vi "UsrProfiles-Save new profile.vi"() -> ()   [LabVIEW 2020]
uses:
  Typedefs/Which path.ctl
  Globals/gl_UsrProfiles globals.vi
panel:
  out "error out":errorcluster
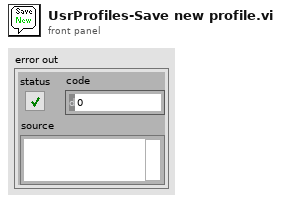
[diagram p1: front panel]
types:
  T1 = typedef "Which path.ctl" = enum16{"Configuration Files", "Calibration Files", "Images", "Setup.ini", "Loaded User profile.ini", "User's-Previous session.ini", "New user profile.ini", "Selected User profile.ini", "User profiles folder", "Power meter scaling.txt", "FOV Cal.ini", "Calibration.ini"}
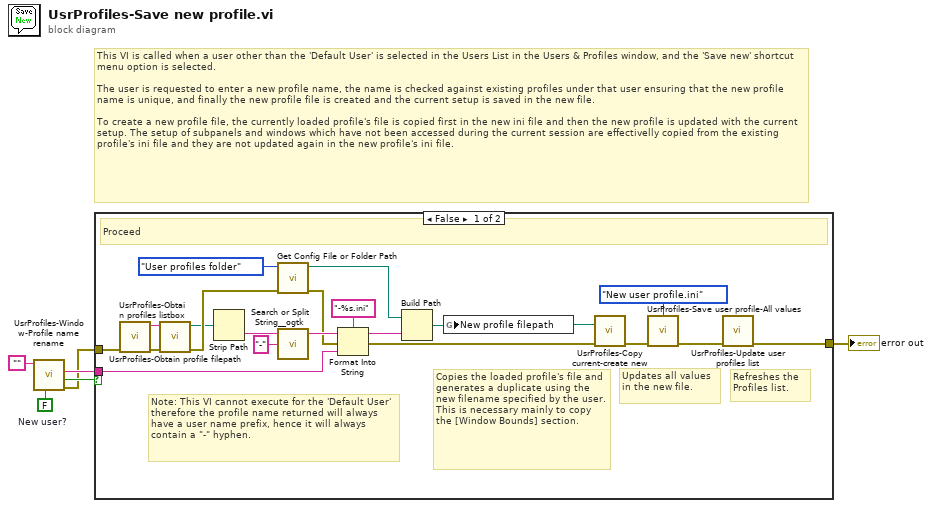
[diagram p0: block diagram]
diagram:
  w1 = FALSE  # New user?
  # "This VI is called when a user other than the 'Default User' is selected in the Users List in the Users & Profiles window, and the 'Save new' shortcut menu option is selected.\n\nThe user is requested to enter a new profile name, the name is checked against existing profiles under that user ensuring that the new profile name is unique, and finally the new profile file is created and the current setup is saved in the new file.\n\nTo create a new profile file, the currently loaded profile's file is copied first in the new ini file and then the new profile is updated with the current setup. The setup of subpanels and windows which have not been accessed during the current session are effectivelly copied from the existing profile's ini file and they are not updated again in the new profile's ini file."
  n1 = call "UsrProfiles-Window-Profile name rename.vi"("New user? (F)"=w1, "Profile name"="") -> ("error out"=w3:errorcluster, "Cancelled (Left button pressed)"=w5:bool, "New profile name"=w4:string)  [unwired: 7 in]
  n2 = case shown="False" w5 {
    tunnel: w4 -> [w19 _]
    tunnel: w3 -> [w14 w27]
    tunnel: [w11 w27] -> w2
    frame False {
      # "Updates all values in the new file."
      # "Copies the loaded profile's file and generates a duplicate using the new filename specified by the user.\nThis is necessary mainly to copy the [Window Bounds] section."
      # "Refreshes the Profiles list."
      # "Note: This VI cannot execute for the 'Default User' therefore the profile name returned will always have a user name prefix, hence it will always contain a \"-\" hyphen."
      # "Proceed"
      n3 = call "UsrProfiles-Obtain profiles listbox.vi"("error in (no error)"=w14) -> ("error out"=w26:errorcluster, "Selected profile's name"=w25:string)  [unwired: 7 in, 2 out]
      n4 = call "UsrProfiles-Obtain profile filepath.vi"("error in"=w26, "Profile name"=w25) -> ("error out"=w16:errorcluster, "Profile filepath"=w7:path)  [unwired: 8 in]
      n5 = Strip Path(path=w7) -> (name=w24:string)  [unwired: 1 out]
      n6 = call "Get Config File or Folder Path.vi"("Error In"=w16, "Which file or folder?"=Which_path."User profiles folder") -> ("Error Out"=w15:errorcluster, "File Path"=w17:path)  [unwired: 7 in, 1 out]
      n7 = call <userlib>:"Search or Split String__ogtk.vi"("search string/char (-)"="-", "string"=w24) -> ("substring before match"=w20:string)  [unwired: 1 in, 2 out]
      n8 = Format Into String(format string="-%s.ini", initial string=w20, error in=w15, w19) -> (resulting string=w18:string, error out=w12:errorcluster)
      n9 = Build Path(base path=w17, name or relative path=w18) -> (appended path=w13:path)
      n10 = global write "gl_UsrProfiles globals.vi" "New profile filepath"(w13) -> ()
      n11 = call "UsrProfiles-Copy current-create new.vi"("error in (no error)"=w12, "New profile's filepath"=w13) -> ("error out"=w9:errorcluster)  [unwired: 9 in]
      n12 = call "UsrProfiles-Save user profile-All values.vi"("error in"=w9, "Which file? (User profile.ini)"=Which_path."New user profile.ini") -> ("error out"=w10:errorcluster)  [unwired: 9 in]
      n13 = call "UsrProfiles-Update user profiles list.vi"("error in"=w10) -> ("error out"=w11:errorcluster)  [unwired: 9 in, 1 out]
    }
    frame True {
      # "Cancelled"
    }
  }
  "error out" <- w2
